vi "Pixel_LIDAR_Close_old.vi"(1 "error in (no error) 2":errorcluster, 2 "Image":T1) -> ()   [LabVIEW 2010]
doc: "This SubVI works with PixelSonar_run and closes down and releases memory after the sonar is run"
uses:
  <vilib>/vision/Image Controls.llb/IMAQ Image.ctl
panel:
  # "This SubVI is designed to close down the PixelSonar_Run.VI and release its memory space"
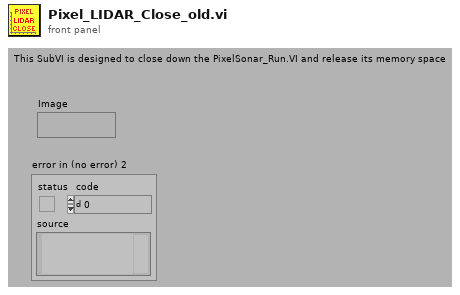
[diagram p1: front panel]
types:
  T1 = typedef "IMAQ Image.ctl" = refnum<image>
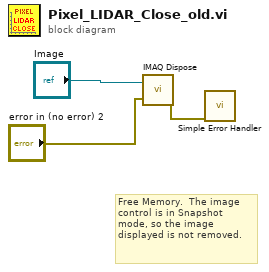
[diagram p0: block diagram]
diagram:
  # "Free Memory.  The image control is in Snapshot mode, so the image displayed is not removed."
  n1 = call "IMAQ Dispose"("Image"="Image", "error in (no error)"="error in (no error) 2") -> ("error out"=w3:errorcluster)  [unwired: 1 in, 3 out]
  n2 = call <vilib>:"Simple Error Handler.vi"("error in (no error)"=w3) -> ()  [unwired: 1 in, 8 out]
